vi "Lab2View.vi"() -> ()   [LabVIEW 2021]
panel:
  out "Received string":string
  in  "String":string
  in  "send":bool
  in  "stop":bool
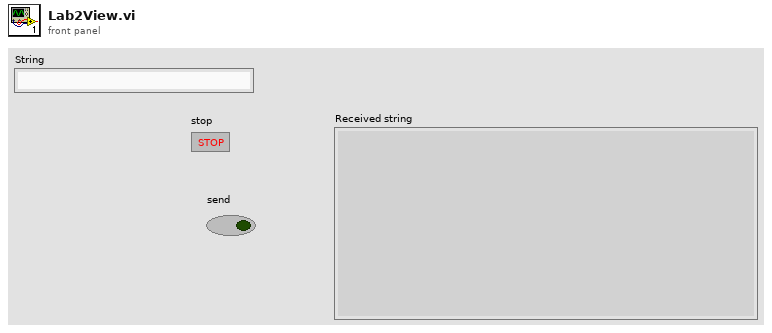
[diagram p1: front panel]
types:
  T1 = enum16{"Standard", "Buffered", "CRLF", "Immediate"}
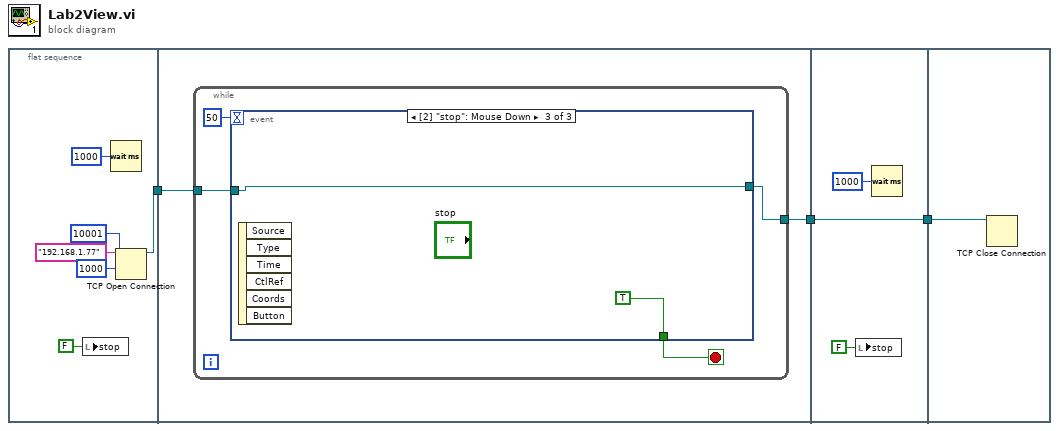
[diagram p0: block diagram]
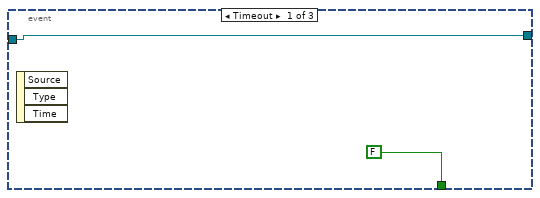
[diagram p2: hidden frame]
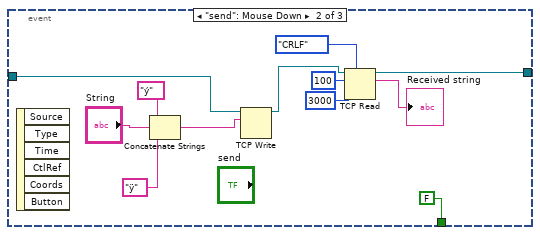
[diagram p3: hidden frame]
diagram:
  n1 = flat-sequence {
    tunnel: [w4] -> w3
    tunnel: w3 -> [w11]
    tunnel: [w10] -> w1
    tunnel: [w32] -> w2
    tunnel: w1 -> [w32]
    tunnel: w2 -> [w35]
    frame #0 {
      n2 = local write "stop"(FALSE ("stop")) -> ()
      n3 = Wait (ms)(milliseconds to wait=u32 1000) -> ()  [unwired: 1 out]
      n4 = TCP Open Connection(address="192.168.1.77", remote port or service name=u16 10001, timeout ms (60000)=1000) -> (connection ID=w4:refnum<k5>)  [unwired: 2 in, 1 out]
    }
    frame #1 {
      n5 = while {
        tunnel: w11 -> [w14]
        tunnel: [w13] -> w10
        stop <- w15 stop-if-true
        n6 = event shown="[2] \"stop\": Mouse Down" {
          selector: _ -> [_ _ _]
          dyn-events: _ -> [_ _ _]
          timeout: 50 -> [_ _ _]
          tunnel: [FALSE FALSE TRUE] -> w15
          tunnel: w14 -> [w16 w20 w30]
          tunnel: [w16 w18 w30] -> w13
          event Timeout {
            n7 = event-data() -> ()  [unwired: 1 in, 3 out]
          }
          event "send": Mouse Down {
            n8 = event-data() -> ()  [unwired: 1 in, 6 out]
            n9 = Concatenate Strings("ý", "String", "ÿ") -> (w26:string)
            n10 = TCP Write(connection ID=w20, data in=w26) -> (connection ID out=w19:refnum<k5>)  [unwired: 2 in, 2 out]
            n11 = TCP Read(connection ID=w19, bytes to read=100, 7:T1."CRLF" ("mode (standard)"), 9:3000 ("timeout ms (25000)")) -> (connection ID out=w18:refnum<k5>, data out=→"Received string":string)  [unwired: 1 in, 1 out]
          }
          event "stop": Mouse Down {
            n12 = event-data() -> ()  [unwired: 1 in, 6 out]
          }
        }
      }
    }
    frame #2 {
      n13 = local write "stop"(FALSE ("stop")) -> ()
      n14 = Wait (ms)(milliseconds to wait=u32 1000) -> ()  [unwired: 1 out]
    }
    frame #3 {
      n15 = TCP Close Connection(connection ID=w35) -> ()  [unwired: 2 in, 2 out]
    }
  }
